vi "Initialize Pin.vi"   [LabVIEW 2021, in "Abstract_Instrument.lvclass"]
doc: "Initialize either a single pin or an array of pins based on the input pins given."
uses:
  Abstract_Instrument.lvclass
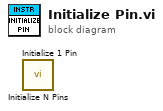
[diagram p0: block diagram]
diagram:
  n1 = call "Initialize N Pins.vi"() -> ()  [unwired: 8 in, 4 out]
  n2 = call "Initialize 1 Pin.vi"() -> ()  [unwired: 8 in, 4 out]
